vi "provide_OME_data.vi"(6 "image ID":string, 8 "error in (no error)":errorcluster, 9 "structuredAttribute string in":string, 10 "OME element in":refnum<class "XMLElement.lvclass">, 11 "GenericScanHead in":refnum<class "GenericScanHead.lvclass">) -> (0 "error out":errorcluster, 1 "structuredAttribute string out":string, 2 "OME element out":refnum<class "XMLElement.lvclass">, 3 "GenericScanHead out":refnum<class "GenericScanHead.lvclass">)   [LabVIEW 2010, in "GenericScanHead.lvclass"]
uses:
  GenericScanHead.lvclass
  common/classes/XMLElement/XMLElement/XMLElement.lvclass
  common/classes/GenericComponent/GenericComponent/GenericComponent.lvclass
  Trajectory/GenericTrajectory/GenericTrajectory/GenericTrajectory.lvclass
  common/classes/ErrorController/ErrorController/class_data.vi
  common/classes/ErrorController/ErrorController/ErrorController.lvclass
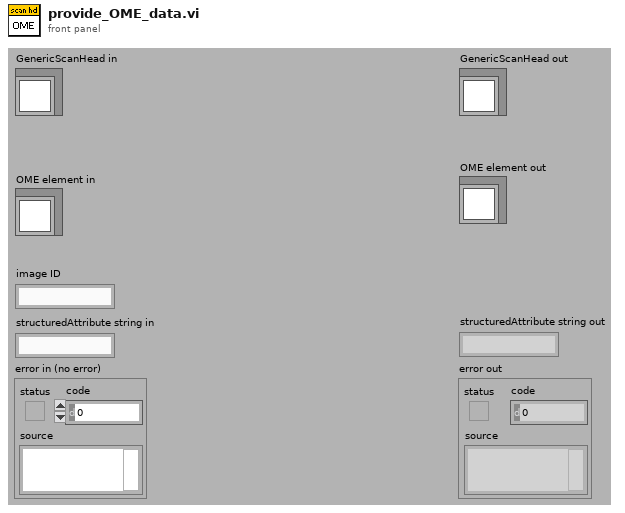
[diagram p1: front panel]
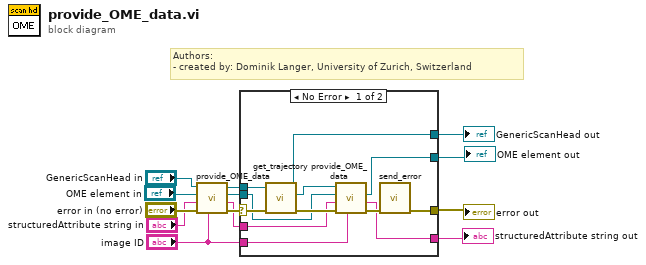
[diagram p0: block diagram]
diagram:
  # "Authors: \n- created by: Dominik Langer, University of Zurich, Switzerland"
  n1 = call-parent "provide_OME_data.vi"("image ID"="image ID", "error in (no error)"="error in (no error)", "structuredAttribute string in"="structuredAttribute string in", "OME element in"="OME element in", "GenericPlugin in"="GenericScanHead in") -> ("error out"=w11:errorcluster, "structuredAttribute string out"=w2:string, "OME element out"=w8:refnum<class "XMLElement.lvclass">, "GenericPlugin out"=w10:refnum<class "GenericScanHead.lvclass">)  [unwired: 3 in]
  n2 = case shown="No Error" w11 {
    selector: w11 -> [w25 w27]
    tunnel: w10 -> [w24 w29]
    tunnel: "image ID" -> [w16 w26]
    tunnel: [w21 w29] -> w9
    tunnel: [w20 w28] -> w5
    tunnel: w8 -> [w19 w28]
    tunnel: [w17 w27] -> w7
    tunnel: w2 -> [w15 _]
    tunnel: [w14 w26] -> w1
    frame No Error {
      n3 = call-dynamic "get_trajectory.vi"("error in (no error)"=w25, "GenericScanHead.lvclass in"=w24) -> ("error out"=w23:errorcluster, "trajectory"=w22:refnum<class "GenericTrajectory.lvclass">, "GenericScanHead.lvclass out"=w21:refnum<class "GenericScanHead.lvclass">)  [unwired: 7 in]
      n4 = call-dynamic "provide_OME_data.vi"("image ID"=w16, "error in (no error)"=w23, "structuredAttribute string in"=w15, "OME element in"=w19, "GenericPlugin in"=w22) -> ("error out"=w18:errorcluster, "structuredAttribute string out"=w14:string, "OME element out"=w20:refnum<class "XMLElement.lvclass">)  [unwired: 3 in, 1 out]
      n5 = call "send_error.vi"("error in (no error)"=w18) -> ("error out"=w17:errorcluster)  [unwired: 10 in]
    }
    frame Error {
    }
  }
  "error out" <- w7
  "GenericScanHead out" <- w9
  "OME element out" <- w5
  "structuredAttribute string out" <- w1
